vi "Set Transfer Byte Order.vi"(8 "error in (no error)":errorcluster, 10 "byte order":T1, 11 "transfer in":T2={"name"="Transfer", "byte order"=enum."big-endian", "settings"=[], "channels"=[]} {"channels"."string offset" format="%d bytes"}) -> (0 "error out":errorcluster, 3 "transfer out":T2={"name"="Transfer", "byte order"=enum."big-endian", "settings"=[], "channels"=[]} {"channels"."string offset" format="%d bytes"})   [LabVIEW 2017, in "DSF Core.lvlib" / "Configuration Session.lvclass"]
uses:
  Configuration Session.lvclass
  Typedefs/DSF Engine Transfer Configuration.ctl
  Typedefs/DSF Byte Order.ctl
  Typedefs/DSF Settings Info.ctl
  Typedefs/DSF Engine Channel Configuration.ctl
  Typedefs/DSF Data Type.ctl
  DSF Core.lvlib
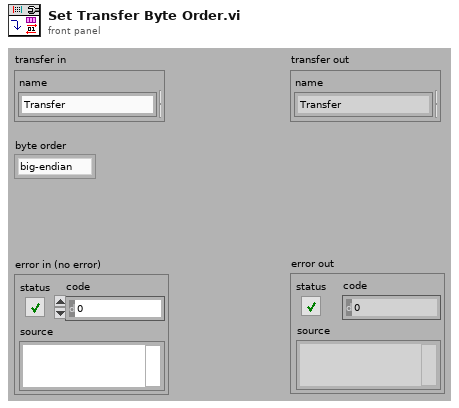
[diagram p1: front panel]
types:
  T1 = typedef "DSF Core.lvlib/DSF Byte Order.ctl" = enum8{"big-endian", "little-endian"}
  T2 = typedef "DSF Core.lvlib/DSF Engine Transfer Configuration.ctl" = cluster{"name":string, "byte order":T1, "settings":T3, "channels":T4[]}
  T3 = typedef "DSF Core.lvlib/DSF Settings Info.ctl" = cluster{"key":string, "value":string}[]
  T4 = typedef "DSF Core.lvlib/DSF Engine Channel Configuration.ctl" = cluster{"string offset":u64, "string data type":T5, "engine data type":T5, "name":string, "settings":T3, "units":string}
  T5 = typedef "DSF Core.lvlib/DSF Data Type.ctl" = enum8{"Bool", "SGL", "DBL", "I8", "I16", "I32", "I64", "U8", "U16", "U32", "U64"}
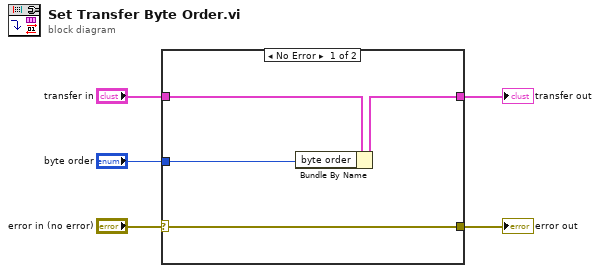
[diagram p0: block diagram]
diagram:
  n1 = case shown="No Error" "error in (no error)" {
    selector: "error in (no error)" -> [w7 w11]
    tunnel: [w7 w11] -> w5
    tunnel: [w8 w10] -> w3
    tunnel: "transfer in" -> [w9 w10]
    tunnel: "byte order" -> [w6 _]
    frame No Error {
      n2 = Bundle By Name(cluster=w9, "byte order"=w6) -> (w8:T2)
    }
    frame Error {
    }
  }
  "error out" <- w5
  "transfer out" <- w3
